vi "setFPGAReference.vi"(10 "FPGAReference":refnum<k20>, 11 "ModbusPort1WriteFIFO in":refnum<class "TimestampUpdateFIFO.lvclass">) -> (3 "ModbusPort1WriteFIFO out":refnum<class "TimestampUpdateFIFO.lvclass">)   [LabVIEW 2016, in "TimestampUpdateFIFO.lvclass"]
uses:
  TimestampUpdateFIFO.lvclass
  TimestampUpdateFIFO.lvclass/TimestampUpdateFIFO.ctl
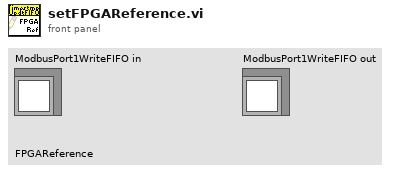
[diagram p1: front panel]
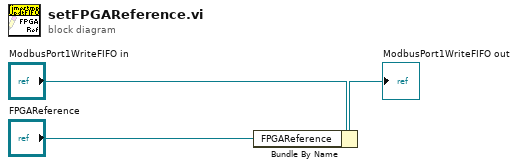
[diagram p0: block diagram]
diagram:
  n1 = Bundle By Name(cluster="ModbusPort1WriteFIFO in", "FPGAReference"="FPGAReference") -> (→"ModbusPort1WriteFIFO out":refnum<class "TimestampUpdateFIFO.lvclass">)
